vi "DAQreset2009.vi"() -> ()   [LabVIEW 2017]
panel:
  out "error out":errorcluster
  in  "stop":bool
  # "This VI Demonstrates how to reset your USB\nDAQ device programmatically if it were to\nbe shut off or unplugged from the system\nNote: You need to open the DAQ assistant\nand make sure to choose the correct device.\n1. Start the VI with your device plugged in\nand working.\n2. Unplug or remove the device and you will\nnotice that it go to the reset loop and waits \nfor device to be reconnected.\nNote: If you want to start with the device\nunplugged you will need to right click the \nDAQ assistant and choose Generate DAQmx\ncode. This will allow you to choose the \nappropriate device prior to starting the VI."
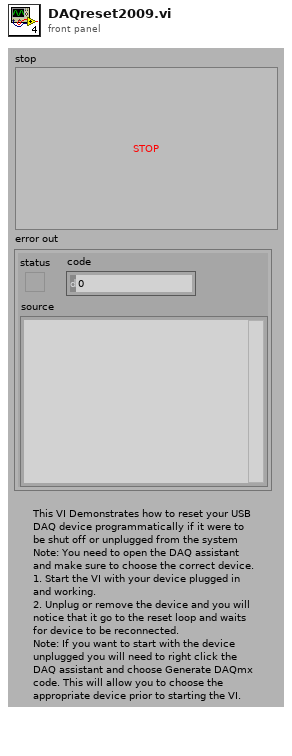
[diagram p1: front panel]
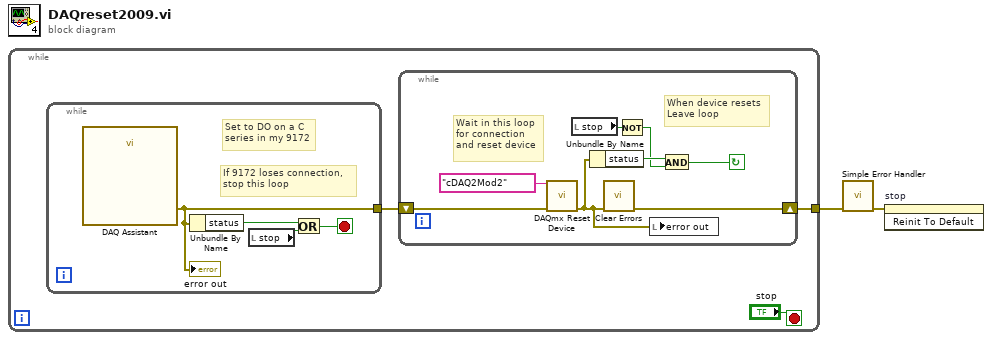
[diagram p0: block diagram]
diagram:
  n1 = while {
    tunnel: [w3] -> w2
    stop <- "stop" stop-if-true
    n2 = while {
      tunnel: [w17] -> w4
      stop <- w15 stop-if-true
      # "If 9172 loses connection, \nstop this loop"
      # "Set to DO on a C\nseries in my 9172"
      n3 = call "DAQ Assistant"() -> ("error out"=w17:errorcluster)  [unwired: 18 in, 1 out]
      "error out" <- w17
      n4 = Unbundle By Name(w17) -> ("status"=w16:bool)
      n5 = local read "stop"() -> (w14:bool)
      n6 = Or(x=w16, y=w14) -> (x .or. y?=w15:bool)
    }
    n7 = while {
      shift-right: [w7] -> w3
      shift-left: w4 -> [w13]
      stop <- w8 continue-if-true
      # "When device resets\nLeave loop"
      # "Wait in this loop\nfor connection\nand reset device"
      n8 = call <vilib>:"DAQmx Reset Device.vi"("device in"=tag "cDAQ2Mod2", "error in"=w13) -> ("error out"=w6:errorcluster)  [unwired: 13 in]
      n9 = local read "stop"() -> (w11:bool)
      n10 = Unbundle By Name(w6) -> ("status"=w10:bool)
      n11 = call <vilib>:"Clear Errors.vi"("error in (no error)"=w6) -> ("error out"=w7:errorcluster)  [unwired: 5 in, 1 out]
      n12 = Not(x=w11) -> (.not. x?=w9:bool)
      n13 = local write "error out"(w6) -> ()
      n14 = And(x=w10, y=w9) -> (x .and. y?=w8:bool)
    }
  }
  n15 = call <vilib>:"Simple Error Handler.vi"("error in (no error)"=w2) -> ("error out"=w1:errorcluster)  [unwired: 4 in, 4 out]
  n16 = invoke on="stop" class="Bool (strict)" method="Reinit To Default"(error in=w1) -> ()  [unwired: 2 in, 3 out]
